vi "Update Parameters Configuration File Error.vi"(8 "error in":errorcluster, 11 "Configuration files Ref":T1 format="%.0x") -> (0 "error out":errorcluster, 3 "Configuration files Ref out":T1 format="%.0x")   [LabVIEW 2020, in "Ballard ARINC 429 System Explorer.lvlib" / "Implementation.lvlib"]
uses:
  Implementation.lvlib
  Scripting/Ballard ARINC 429 Scripting.lvlib
  <vilib>/NI VeriStand/Custom Device API/Custom Device API.lvlib
  <vilib>/NI VeriStand/Custom Device API/Get Item Property (Boolean).vi
  Scripting/Constants.vi
  <vilib>/NI VeriStand/Custom Device API/Custom Device Item Ref.ctl
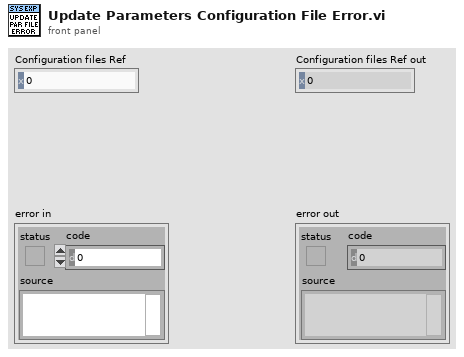
[diagram p1: front panel]
types:
  T1 = typedef "Custom Device API.lvlib/Custom Device Item Ref.ctl" = u64
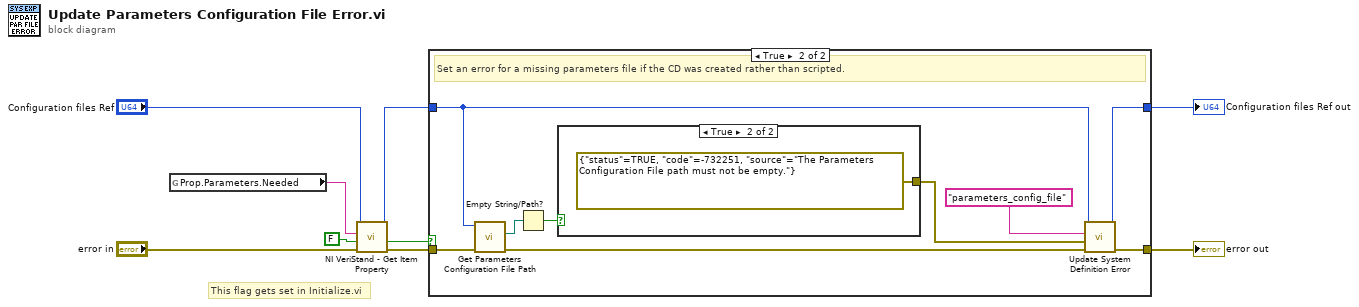
[diagram p0: block diagram]
diagram:
  # "This flag gets set in Initialize.vi"
  n1 = global read "Constants.vi" "Prop.Parameters.Needed"() -> (w1:string)
  n2 = call-poly <vilib>:"NI VeriStand - Get Item Property.vi"("error in (no error)"="error in", "Default Value"=FALSE, "Property Name"=w1, "Item Ref in"="Configuration files Ref") -> ("error out"=w5:errorcluster, "Value"=w7:bool, "Item Ref out"=w3:T1)  [unwired: 4 in, 1 out]
  n3 = case shown="True" w7 {
    tunnel: [w10 w20] -> w9
    tunnel: [w11 w19] -> w8
    tunnel: w5 -> [w11 w18]
    tunnel: w3 -> [w10 w12]
    frame False {
      # "Parameters configuration file is not needed if the CD was scripted."
    }
    frame True {
      # "Set an error for a missing parameters file if the CD was created rather than scripted."
      n4 = call "Get Parameters Configuration File Path.vi"("error in"=w18, "Configuration files Ref"=w12) -> ("error out"=w16:errorcluster, "Path"=w13:path)  [unwired: 7 in, 1 out]
      n5 = Empty String/Path?(string/path=w13) -> (empty?=w17:bool)
      n6 = case shown="True" w17 {
        tunnel: [_ errorcluster {"status"=TRUE, "code"=-732251, "source"="The Parameters Configuration File path must not be empty."} ("New Error")] -> w15
        frame False {
        }
        frame True {
        }
      }
      n7 = call "Update System Definition Error.vi"("error to report"=w16, "error in"=w15, "error key"="parameters_config_file", "Configuration files Ref"=w12) -> ("error out"=w19:errorcluster, "Configuration files Ref out"=w20:T1)  [unwired: 6 in]
    }
  }
  "error out" <- w8
  "Configuration files Ref out" <- w9
